vi "SetWaveformXscale.vi"(7 "Plot Duration":dbl=15.0 format="%#_13g", 10 "deltaT":dbl, 11 "WaveformChart in":refnum<vi>) -> ()   [LabVIEW 2013]
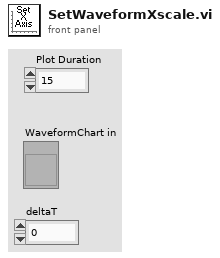
[diagram p1: front panel]
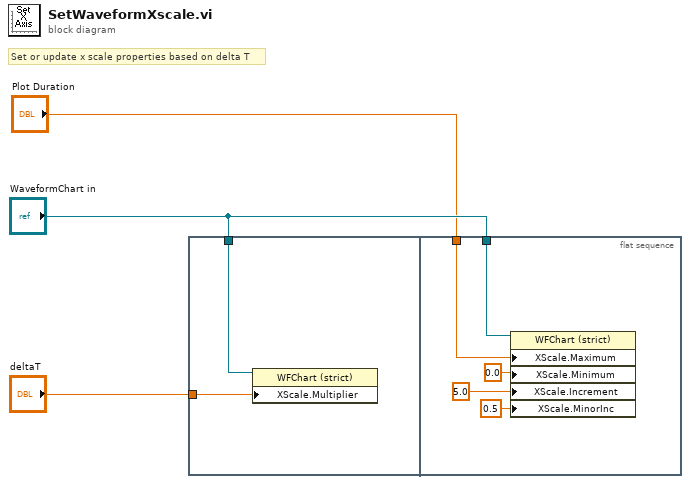
[diagram p0: block diagram]
diagram:
  # "Set or update x scale properties based on delta T"
  n1 = flat-sequence {
    tunnel: "deltaT" -> [w5]
    tunnel: "WaveformChart in" -> [w4]
    tunnel: "WaveformChart in" -> [w9]
    tunnel: "Plot Duration" -> [w6]
    frame #0 {
      n2 = property on="Property Node" class="WFChart (strict)"(reference=w4, "XScale.Multiplier"=w5) -> ()  [unwired: 1 in, 2 out]
    }
    frame #1 {
      n3 = property on="Property Node" class="WFChart (strict)"(reference=w9, "XScale.Maximum"=w6, "XScale.Minimum"=0.0 ("X Scale.Range:Minimum"), "XScale.Increment"=5.0 ("X Scale.Range:Increment"), "XScale.MinorInc"=0.5 ("X Scale.Range:Minor Increment")) -> ()  [unwired: 1 in, 2 out]
    }
  }
